vi "QPMX Close.vi"(8 "error in":errorcluster, 11 "QPMX ssn":T1={"visa"="", "switch mode"=enum."Switched by TWM", "sequence"=[], "timing delays"=[], "polarity"=enum."Positive", "ss delay (s)"=2.0, "internal timer (s)"=1.0, "Last loaded sequence file"=path ""} {"internal timer (s)" min=0.0 step=1.0; "ss delay (s)" min=0.0 step=1.0; "timing delays" min=1 max=255 step=1}) -> (0 "error out":errorcluster)   [LabVIEW 2020]
doc: "Wrapper layer between TWM and QuPMXdriver. Close multiplexer."
uses:
  Generic COM/QPMX Session.ctl
  QPMX switch mode.ctl
  QPMX polarity.ctl
  QuPMXLabVIEWdriver/QuPMXdriver.lvlib
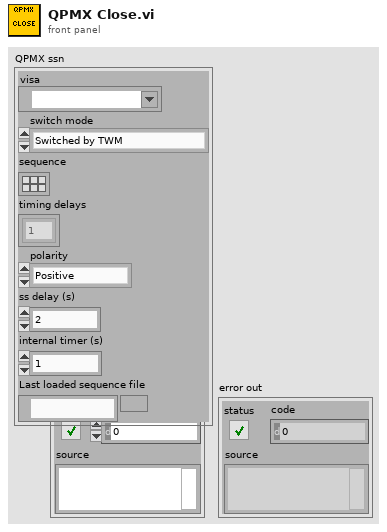
[diagram p1: front panel]
types:
  T1 = typedef "QPMX Session.ctl" = cluster{"visa":refnum<visa-resource-name>, "switch mode":T2, "sequence":bool[][], "timing delays":u32[], "polarity":T3, "ss delay (s)":dbl, "internal timer (s)":dbl, "Last loaded sequence file":path}
  T2 = typedef "QPMX switch mode.ctl" = enum16{"Switched by TWM", "Switched by external clock", "Switched by internal clock"}
  T3 = typedef "QPMX polarity.ctl" = enum16{"Positive", "Negative"}
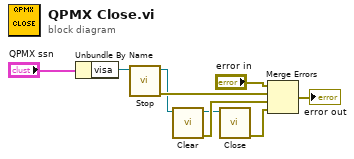
[diagram p0: block diagram]
diagram:
  n1 = Unbundle By Name("QPMX ssn") -> ("visa"=w5:refnum<visa-resource-name>)
  n2 = call "Stop.vi"("VISA resource name"=w5) -> ("error out"=w4:errorcluster, "VISA resource name out"=w3:refnum<visa-resource-name>)  [unwired: 9 in]
  n3 = call "Clear.vi"("VISA resource name"=w3) -> ("error out"=w2:errorcluster, "VISA resource name out"=w1:refnum<visa-resource-name>)  [unwired: 9 in]
  n4 = call "Close.vi"("VISA resource name"=w1) -> ("error out"=w6:errorcluster)  [unwired: 10 in]
  n5 = Merge Errors("error in", w4, w2, w6) -> (→"error out":errorcluster)
